vi "Update-pane-reference.vi"(8 "error in (no error)":errorcluster, 10 "Sorted pane references":refnum<vi>[](array[refnum]), 11 "Pane in":T1) -> (0 "error out":errorcluster, 3 "Pane out":T1)   [LabVIEW 2013, in "PaneToggle.lvlib" / "Panes.lvclass"]
uses:
  Panes.lvclass
  Pane-settings.ctl
  Pane-names.ctl
  Splitter-settings.ctl
  Splitter-names.ctl
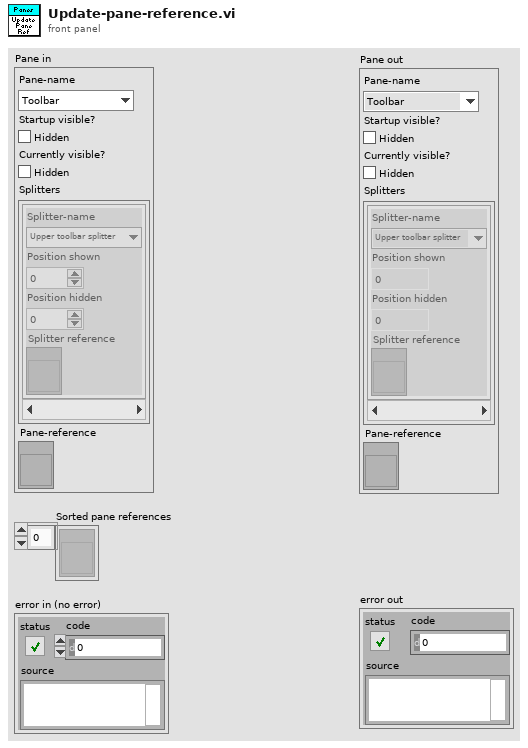
[diagram p1: front panel]
types:
  T1 = typedef "PaneToggle.lvlib/Panes.lvclass/Pane-settings.ctl" = cluster{"Pane-name":T2, "Startup visible?":bool, "Currently visible?":bool, "Splitters":T3[], "Pane-reference":refnum<vi>}
  T2 = typedef "PaneToggle.lvlib/Panes.lvclass/Pane-names.ctl" = enum16{"Toolbar", "Help bar", "Toolbar lower border", "Main panel", "Status bar upper border", "General state bar", "Information bar"}
  T3 = typedef "PaneToggle.lvlib/Panes.lvclass/Splitter-settings.ctl" = cluster{"Splitter-name":T4, "Position shown":i32, "Position hidden":i32, "Splitter reference":refnum<vi>}
  T4 = typedef "PaneToggle.lvlib/Panes.lvclass/Splitter-names.ctl" = enum16{"Upper toolbar splitter", "Help bar splitter", "Lower toolbar splitter", "Upper status bar splitter", "Lower status bar splitter", "Left status bar splitter"}
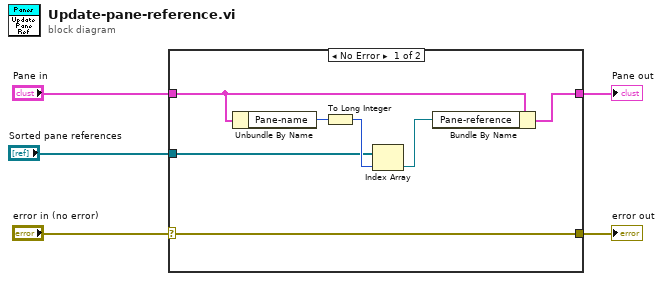
[diagram p0: block diagram]
diagram:
  n1 = case shown="No Error" "error in (no error)" {
    selector: "error in (no error)" -> [w6 w13]
    tunnel: [w12 w14] -> w5
    tunnel: "Pane in" -> [w10 w14]
    tunnel: "Sorted pane references" -> [w8 _]
    tunnel: [w6 w13] -> w1
    frame No Error {
      n2 = Unbundle By Name(w10) -> ("Pane-name"=w7:T2)
      n3 = To Long Integer(number=w7) -> (32bit integer=w9:i32)
      n4 = Index Array(array=w8, index=w9) -> (element=w11:refnum<vi>)
      n5 = Bundle By Name(cluster=w10, "Pane-reference"=w11) -> (w12:T1)
    }
    frame Error {
    }
  }
  "error out" <- w1
  "Pane out" <- w5
